vi "Read Continuous B Sweep.json.vi"(8 "error in (no error)":errorcluster, 10 "file (use dialog)":path, 11 "SweepControl in":refnum<class "SweepControl.lvclass">) -> (0 "error out":errorcluster, 3 "SweepControl out":refnum<class "SweepControl.lvclass">)   [LabVIEW 2016, in "SweepControl.lvclass"]
uses:
  SweepControl.lvclass
  Typedefs/Continuous B Sweep Configuration--Cluster.ctl
  Typedefs/Enum - Experiments.ctl
  Control Experiment/Typedefs/Experiment Description--cluster.ctl
  Control Experiment/Typedefs/Instrument--enum.ctl
  <userlib>/_OpenG.lib/dictionary/dictionary.llb/Dictionary Object RefNum__ogtk.ctl
  <userlib>/_OpenG.lib/dictionary/dictionary.llb/Dictionary Object RefNum - Enum__ogtk.ctl
  Control Experiment/Typedefs/Wiring Description--cluster.ctl
  <userlib>/LevyLab/Lockin-Multichannel/LockinDAQ/Typedefs/AO-cluster.ctl
  <userlib>/LevyLab/Lockin-Multichannel/LockinDAQ/Typedefs/Function-enum.ctl
  <userlib>/LevyLab/Lockin-Multichannel/LockinDAQ/Typedefs/REF-cluster.ctl
  <userlib>/LevyLab/Krohn Hite 7008/typedefs/KH_control_array.ctl
  <userlib>/LevyLab/Krohn Hite 7008/typedefs/KH_control.ctl
  <userlib>/LevyLab/Krohn Hite 7008/typedefs/Channel-Enum.ctl
  <userlib>/LevyLab/Krohn Hite 7008/typedefs/Gain-Enum.ctl
  <userlib>/LevyLab/Krohn Hite 7008/typedefs/Shunt-Enum.ctl
  <userlib>/LevyLab/Krohn Hite 7008/typedefs/Input Configuration-Enum.ctl
  <vilib>/addons/_JKI.lib/Serialization/JSON/JKI JSON Serialization.lvlib
  <userlib>/LevyLab/Krohn Hite 7008/Instrument.KH7008.lvclass
  <userlib>/LevyLab/Lockin-Multichannel/LockinDAQ/LockinDAQ.lvclass
  Control Experiment/Control Experiment.lvclass
panel:
  out "ContinuousBSweep":T1 {"Lockin"."Channels: Lockin"."order" min=1; "Lockin"."Channels: Lockin"."TC (s)" min=1e-05 format="%#_3p"; "Lockin"."Channels: Lockin"."Phase (°)" format="%.3g"; "Lockin"."Channels: Lockin"."f (Hz)" format="%.3g"; "Lockin"."Channels: AO"."f (Hz)" min=0.001 max=10000.0 format="%.3g"; "Lockin"."Channels: AO"."Phase (°)" format="%.3g"; "Lockin"."Channels: AO"."DC (V)" format="%.3p"; "Lockin"."Channels: AO"."Amp (V)" min=0.0 max=10.0 format="%.3p"}
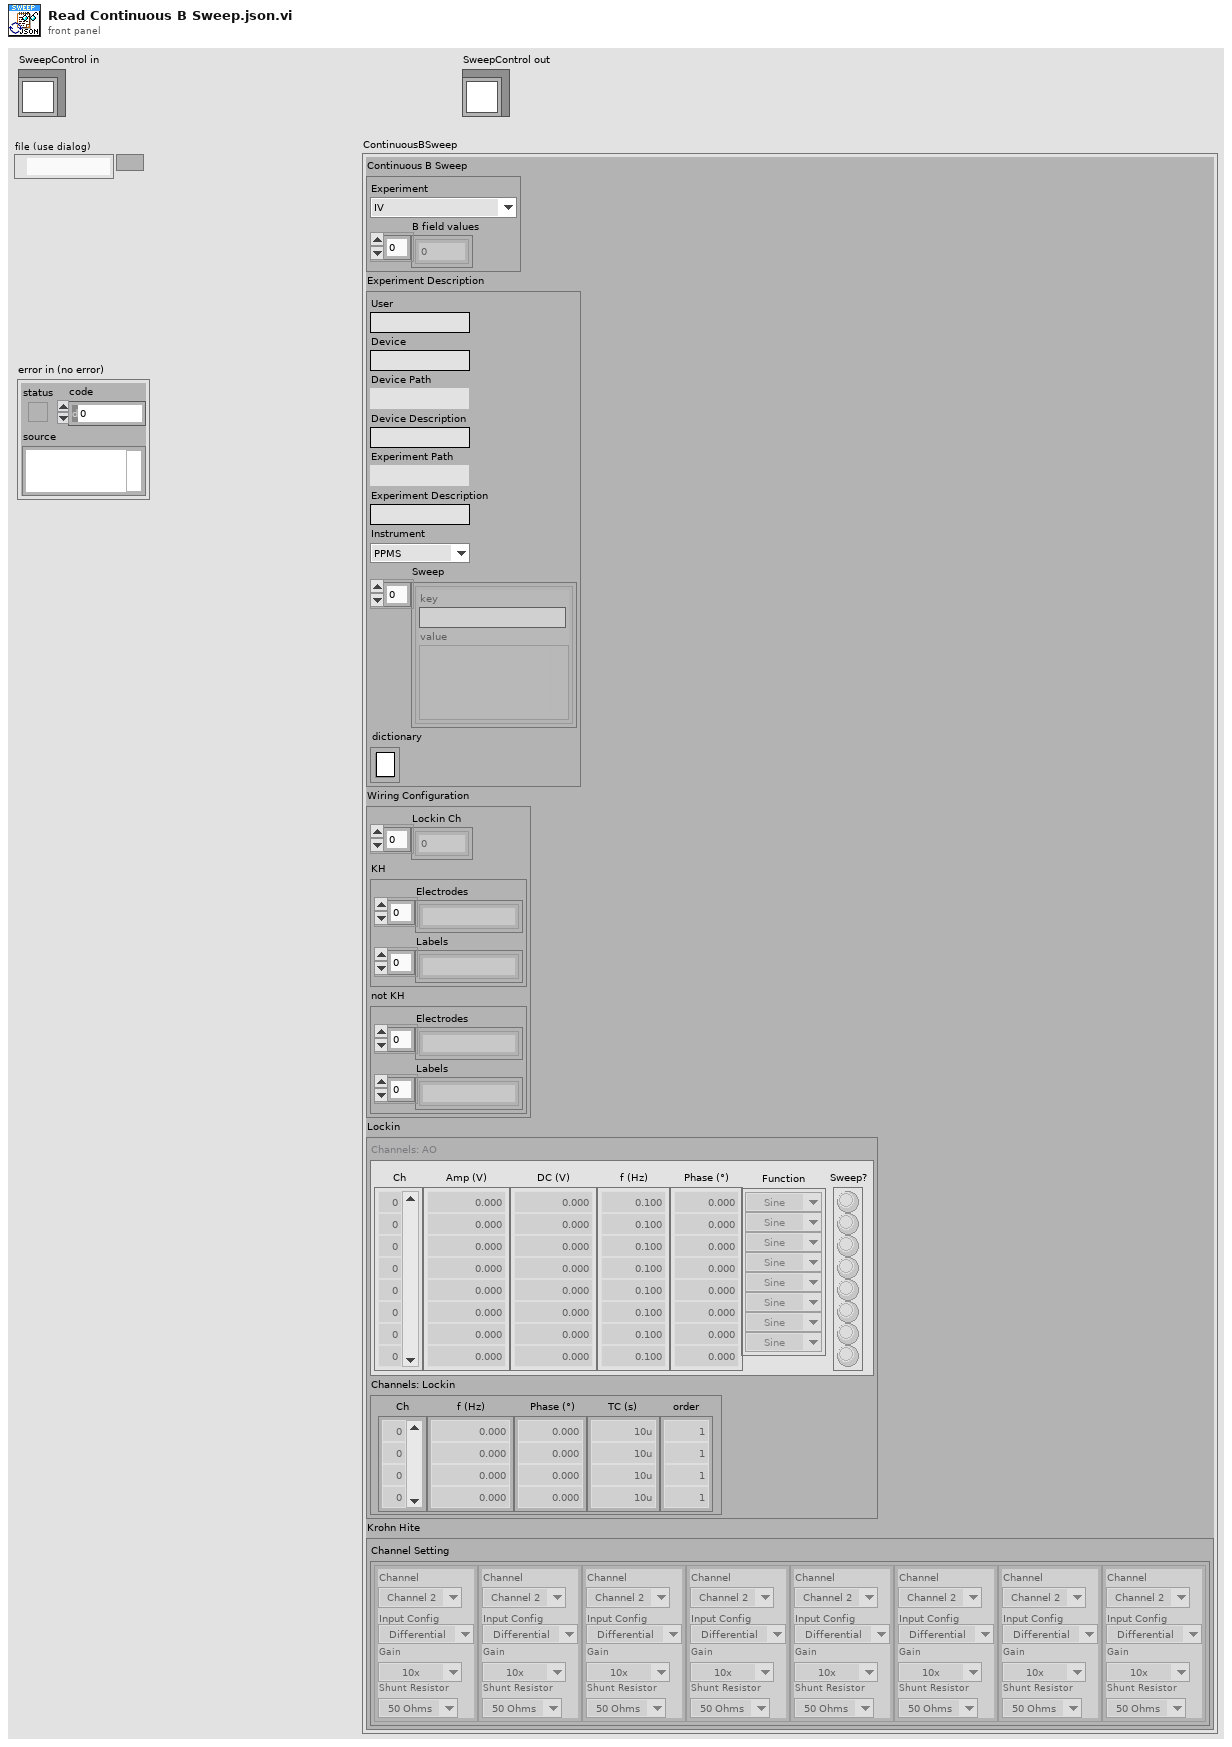
[diagram p1: front panel]
types:
  T1 = typedef "SweepControl.lvclass/Continuous B Sweep Configuration--Cluster.ctl" = cluster{"Continuous B Sweep":cluster{"Experiment":T2, "B field values":dbl[]}, "Experiment Description":T3, "Wiring Configuration":T6, "Lockin":cluster{"Channels: AO":T7, "Channels: Lockin":T9}, "Krohn Hite":cluster{"Channel Setting":T10}}
  T2 = typedef "SweepControl.lvclass/Enum - Experiments.ctl" = enum16{"IV", "IV_Fast", "IV_Sweep", "THz_DelayLine", "Lockin_Vsg", "Lockin_Sweep", "Lockin_Time", "AI WFM time", "Lockin (experimental)"}
  T3 = typedef "Control Experiment.lvclass/Experiment Description--cluster.ctl" = cluster{"User":string, "Device":string, "Device Path":path, "Device Description":string, "Experiment Path":path, "Experiment Description":string, "Instrument":T4, "Sweep":cluster{"key":string, "value":variant}[], "dictionary":T5}
  T4 = typedef "Control Experiment.lvclass/Instrument--enum.ctl" = enum16{"PPMS", "PPMS2", "DR200", "MNK", "CF900", "MFP3D", "CYPHER", "AGILENT", "JEOL", "THz1", "THz2", "EBL"}
  T5 = typedef "Dictionary Object RefNum__ogtk.ctl" = refnum<k1>
  T6 = typedef "Control Experiment.lvclass/Wiring Description--cluster.ctl" = cluster{"Lockin Ch":i32[], "KH":cluster{"Electrodes":string[], "Labels":string[]}, "not KH":cluster{"Electrodes":string[], "Labels":string[]}}
  T7 = typedef "LockinDAQ.lvclass/AO-cluster.ctl" = cluster{"Ch":i32[], "Amp (V)":dbl[], "DC (V)":dbl[], "f (Hz)":dbl[], "Phase (°)":dbl[], "Function":T8[], "Sweep?":bool[]}
  T8 = typedef "LockinDAQ.lvclass/Function-enum.ctl" = enum16{"Sine", "Triangle", "Square", "Sawtooth"}
  T9 = typedef "LockinDAQ.lvclass/REF-cluster.ctl" = cluster{"Ch":i32[], " f (Hz)":dbl[], "Phase (°)":dbl[], "TC (s)":dbl[], "order":i32[]}
  T10 = typedef "Instrument.KH7008.lvclass/KH_control_array.ctl" = T11[]
  T11 = typedef "Instrument.KH7008.lvclass/KH_control.ctl" = cluster{"Channel":T12, "Gain":T13, "Shunt Resistor":T14, "Input Config":T15}
  T12 = typedef "Instrument.KH7008.lvclass/Channel-Enum.ctl" = enum16{"Channel 1", "Channel 2", "Channel 3", "Channel 4", "Channel 5", "Channel 6", "Channel 7", "Channel 8"}
  T13 = typedef "Instrument.KH7008.lvclass/Gain-Enum.ctl" = enum16{"1x", "10x", "100x", "1000x"}
  T14 = typedef "Instrument.KH7008.lvclass/Shunt-Enum.ctl" = enum16{"Open", "50 Ohms", "500 Ohms", "5k Ohms", "50k Ohms"}
  T15 = typedef "Instrument.KH7008.lvclass/Input Configuration-Enum.ctl" = enum16{"Ground", "SE+ (-gnd)", "SE- (+gnd)", "Differential"}
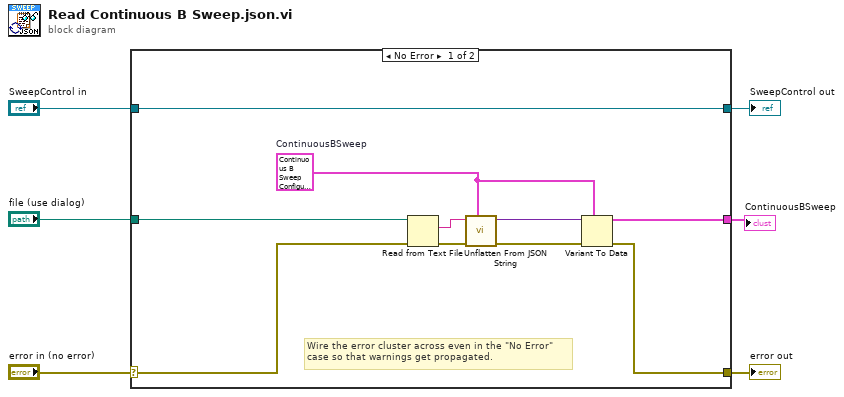
[diagram p0: block diagram]
diagram:
  n1 = case shown="No Error" "error in (no error)" {
    selector: "error in (no error)" -> [w13 w18]
    tunnel: [w11 w18] -> w5
    tunnel: [w16 w17] -> w3
    tunnel: "SweepControl in" -> [w16 w17]
    tunnel: "file (use dialog)" -> [w9 _]
    tunnel: [w8 _] -> w1
    frame No Error {
      w7 = T1 {"Continuous B Sweep"={"Experiment"=enum."IV", "B field values"=[]}, "Experiment Description"={"User"="", "Device"="", "Device Path"=path "", "Device Description"="", "Experiment Path"=path "", "Experiment Description"="", "Instrument"=enum."PPMS", "Sweep"=[], "dictionary"=refnum}, "Wiring Configuration"={"Lockin Ch"=[], "KH"={"Electrodes"=[], "Labels"=[]}, "not KH"={"Electrodes"=[], "Labels"=[]}}, "Lockin"={"Channels: AO"={"Ch"=[], "Amp (V)"=[], "DC (V)"=[], "f (Hz)"=[], "Phase (°)"=[], "Function"=[], "Sweep?"=[]}, "Channels: Lockin"={"Ch"=[], " f (Hz)"=[], "Phase (°)"=[], "TC (s)"=[], "order"=[]}}, "Krohn Hite"={"Channel Setting"=[]}}  # ContinuousBSweep
      # "Wire the error cluster across even in the \"No Error\"\ncase so that warnings get propagated."
      n2 = Read from Text File(file (use dialog)=w9, error in=w13) -> (text=w14:string, error out=w15:errorcluster)  [unwired: 2 in, 2 out]
      n3 = call <vilib>:"Unflatten From JSON String.vi"("Type and Defaults"=w7, "error in (no error)"=w15, "JSON String"=w14) -> ("error out"=w12:errorcluster, "Variant"=w10:variant)  [unwired: 7 in]
      n4 = Variant To Data(error in=w12, type=w7, Variant=w10) -> (data=w8:T1, error out=w11:errorcluster)
    }
    frame Error {
    }
  }
  "error out" <- w5
  "SweepControl out" <- w3
  "ContinuousBSweep" <- w1
